vi "LoadProjectData.vi"(8 "error in (no error)":errorcluster, 11 "MPC_AutoPast in":refnum<class "MPC_AutoInspection.lvclass">) -> (0 "error out":errorcluster, 3 "MPC_AutoPast out":refnum<class "MPC_AutoInspection.lvclass">)   [LabVIEW 2019, in "MPC_AutoInspection.lvclass"]
uses:
  MPC_AutoInspection.lvclass
  LLB/Commonly VI/Ctrl/IDLevel.ctl
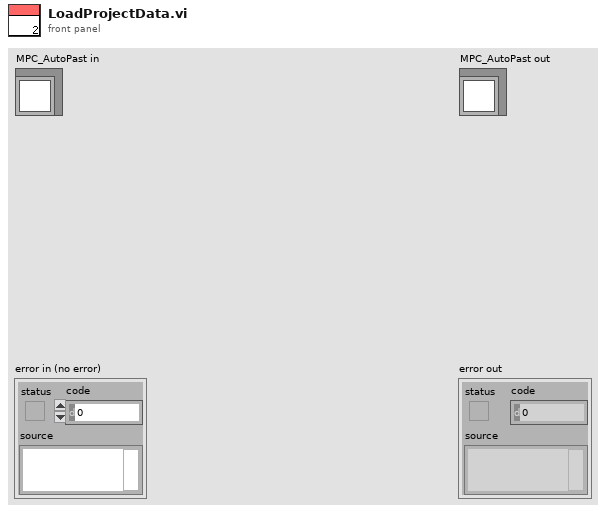
[diagram p1: front panel]
types:
  T1 = enum16{"initial", "save", "load", "write", "read"}
  T2 = enum8{"Enabled", "Disabled", "Disabled and Grayed Out"}
  T3 = typedef "IDLevel.ctl" = enum16{"Administrator", "Engineer", "Operator", "LogIn/Out"}
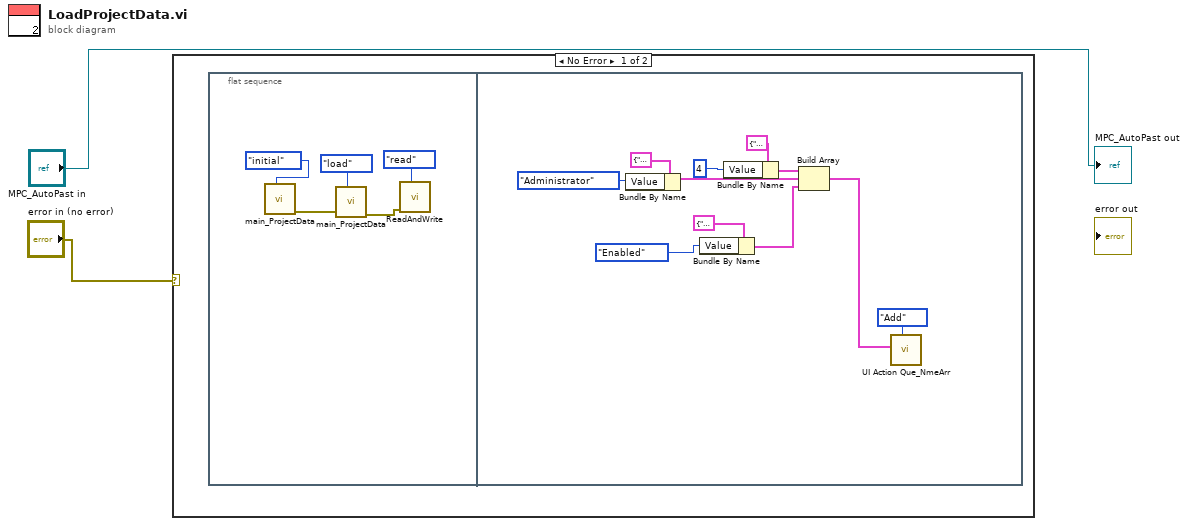
[diagram p0: block diagram]
diagram:
  n1 = case shown="No Error" "error in (no error)" {
    frame No Error {
      n2 = flat-sequence {
        frame #0 {
          n3 = call "main_ProjectData.vi"("Enum"=T1."initial") -> ("error out"=w3:errorcluster)  [unwired: 8 in, 2 out]
          n4 = call "main_ProjectData.vi"("Enum"=T1."load", "error in"=w3) -> ("error out"=w7:errorcluster)  [unwired: 7 in, 2 out]
          n5 = call "ReadAndWrite.vi"("Enum"=enum16{"initial", "save", "read"}."read", "error in"=w7) -> ()  [unwired: 9 in, 1 out]
        }
        frame #1 {
          n6 = Bundle By Name(cluster=cluster{"Action":string, "Value":variant} {"Action"="ChangeMenuBar", "Value"=variant} ("UI Action"), "Value"=IDLevel."Administrator" ("Entry Level")) -> (w11:cluster{"Action":string, "Value":variant})
          n7 = Bundle By Name(cluster=cluster{"Action":string, "Value":variant} {"Action"="AutorunEnable", "Value"=variant} ("UI Action"), "Value"=T2."Enabled" ("Disabled")) -> (w9:cluster{"Action":string, "Value":variant})
          n8 = Bundle By Name(cluster=cluster{"Action":string, "Value":variant} {"Action"="ChangePage", "Value"=variant} ("UI Action"), "Value"=4) -> (w16:cluster{"Action":string, "Value":variant})
          n9 = Build Array(w16, w11, w9) -> (w15:cluster{"Action":string, "Value":variant}[])
          n10 = call "UI Action Que_NmeArr.vi"("Action"=enum16{"Initial", "Add", "Release"}."Add", "UI Process"=w15) -> ()  [unwired: 8 in, 2 out]
        }
      }
    }
    frame Error {
    }
  }
  "MPC_AutoPast out" <- "MPC_AutoPast in"
